vi "ConcatanateFiles.vi"() -> ()   [LabVIEW 2018]
uses:
  <vilib>/Utility/file.llb/Write Delimited Spreadsheet (string).vi
  <vilib>/Utility/file.llb/Read Delimited Spreadsheet (string).vi
panel:
  in  "Combo Box":string(combo)
  in  "path":path=path "C:/RageATE Results/Files to Process"
  out "OutputFile":string="REV-B_TETRA_RX-DVT-Quick_SN_0033_032922-100611_Concat.csv"
  out "Array":string[][](array[string])=[["25", "18.75", "1.000000", "5", "-73", "-1", "-1", "20.000000", "0.577759", "10.832978", "2", "0", "2", "2", "2", "2", "9.995", "10", "-41.21", "31.79", "9.965804", "-39.098881", "-57.496654", "18.397772", "9.965804", "11.713346", "18.311", "0.998", "0.996", "1.807", "3.315", "1.196", "4.993", "3.316", "2.496", "2.516", "3.568", "5.472", "2.824", "2.888", "2.336", "1.448", "0.284", "0.128", "0.686", "0.3", "1.225", "1.12", "24.977425", "25.191151", "27.1", "33", "30.875", "32.25", "31.625", "31.125", "20000", "-41.009443", "136.150678", "1", "0", "3/29/2022 11:45:52 AM", "P0033", "-1", "-1", "adcsync -vADC ERR: 255 255 255 255loop retry_limit_ms 10000...ADC ERR: 255 255 255 255loop retry_limit_ms 9980...ADC ERR: 000 000 000 000ADC ERR: 000 000 000 000ADC ERR: 000 000 000 000ADC ERR: 000 000 000 000ADC ERR: 000 000 000 000ADC ERR: 000 000 000 000ADC ERR: 000 000 000 000ADC ERR: 000 000 000 000ADC0 Frame: 0x30AAA555AAA55500 <- VALIDADC1 Frame: 0x31AAA555AAA55500 <- VALIDADC2 Frame: 0x32AAA555AAA55500 <- VALIDADC3 Frame: 0x33AAA555AAA55500 <- VALIDend retry_limit_ms 9890ADCSYNC PASSED>", "-1", "4F 4F CE CE", "0", "1", "18.000000", "5.000000", "50.000000", "30.000000", "15.000000", "0.000000", "111", "1"], ["25", "18.75", "1.000000", "5", "-73", "-1", "-1", "25.000000", "0.566155", "10.615412", "2", "0", "2", "2", "2", "2", "12.495", "10", "-34.244", "38.756", "9.965804", "-32.195411", "-56.557369", "24.361958", "9.965804", "5.686631", "18.311", "0.997", "0.997", "1.808", "3.317", "1.195", "4.99", "3.316", "2.497", "2.519", "3.56", "5.472", "2.832", "2.888", "2.336", "1.448", "0.29", "0.128", "0.669", "0.291", "1.226", "1.121", "24.97603", "25.195795", "26.05", "33.125", "30.875", "32.125", "31.875", "31.125", "25000", "-41.697643", "10.598856", "2", "1", "3/29/2022 11:46:03 AM", "P0033", "-1", "-1", "-1", "-1", "30 31 32 33", "1", "-1", "18.000000", "5.000000", "50.000000", "30.000000", "8.000000", "0.000000", "111", "1"], ["25", "18.75", "1.000000", "5", "-73", "-1", "-1", "30.000000", "0.56922", "10.672877", "3", "0", "2", "2", "2", "2", "14.995", "10", "-35.696", "37.304", "9.965804", "-33.635349", "-59.768319", "26.13297", "9.965804", "3.927681", "18.311", "0.997", "0.995", "1.807", "3.316", "1.194", "4.992", "3.316", "2.497", "2.516", "3.568", "5.472", "2.824", "2.888", "2.336", "1.448", "0.289", "0.127", "0.689", "0.295", "1.228", "1.155", "24.977425", "25.19043", "28.15", "33", "30.75", "32.375", "31.875", "31.25", "30000", "-42.531268", "11.002014", "3", "1", "3/29/2022 11:46:14 AM", "P0033", "-1", "-1", "-1", "-1", "30 31 32 33", "1", "-1", "18.000000", "5.000000", "50.000000", "30.000000", "6.500000", "0.000000", "111", "1"], ["25", "18.75", "1.000000", "5", "-73", "-1", "-1", "35.000000", "0.567535", "10.641274", "3", "0", "2", "2", "2", "2", "17.495", "10", "-42.928", "30.072", "9.965804", "-40.790008", "-63.593921", "22.803913", "9.965804", "7.334079", "18.329", "0.997", "0.994", "1.807", "3.315", "1.196", "4.992", "3.314", "2.496", "2.516", "3.568", "5.472", "2.824", "2.888", "2.336", "1.448", "0.282", "0.127", "0.684", "0.292", "1.226", "1.117", "24.975447", "25.132133", "27.1", "32.875", "31", "32.375", "31.75", "31.125", "35000", "-41.740204", "10.999033", "4", "1", "3/29/2022 11:46:25 AM", "P0033", "-1", "-1", "-1", "-1", "30 31 32 33", "1", "-1", "18.000000", "5.000000", "50.000000", "30.000000", "9.000000", "0.000000", "111", "1"], ["25", "18.75", "1.000000", "5", "-73", "-1", "-1", "40.000000", "0.559301", "10.486896", "3", "0", "2", "2", "2", "2", "19.995", "10", "-45.764", "27.236", "9.965804", "-43.646918", "-66.38804", "22.741122", "9.965804", "7.37596", "18.32", "0.997", "0.996", "1.808", "3.314", "1.194", "4.989", "3.317", "2.498", "2.516", "3.568", "5.472", "2.832", "2.896", "2.336", "1.456", "0.284", "0.128", "0.657", "0.278", "1.227", "1.141", "24.976114", "25.126818", "26.05", "33.125", "30.75", "32.375", "31.75", "31.25", "40000", "-43.030043", "10.904585", "5", "1", "3/29/2022 11:46:36 AM", "P0033", "-1", "-1", "-1", "-1", "30 31 32 33", "1", "-1", "18.000000", "5.000000", "50.000000", "30.000000", "10.000000", "0.000000", "101", "0"], ["25", "18.75", "2.000000", "5", "-73", "-1", "-1", "20.000000", "0.570127", "10.689885", "2", "0", "2", "2", "2", "2", "9.995", "10", "-39.777", "33.223", "9.965804", "-37.717005", "-57.015434", "19.298429", "9.965804", "10.761566", "18.32", "0.998", "0.995", "1.807", "3.315", "1.196", "4.992", "3.318", "2.496", "2.517", "3.568", "5.472", "2.824", "2.888", "2.336", "1.448", "0.282", "0.128", "0.686", "0.3", "1.226", "1.121", "24.976858", "25.185183", "27.1", "33", "31", "32.375", "31.875", "31.125", "20000", "-41.009443", "14.075206", "6", "1", "3/29/2022 11:46:50 AM", "P0033", "-1", "-1", "-1", "-1", "30 31 32 33", "1", "-1", "18.000000", "5.000000", "50.000000", "30.000000", "15.000000", "0.000000", "111", "1"], ["25", "18.75", "2.000000", "5", "-73", "-1", "-1", "25.000000", "0.566302", "10.618161", "2", "0", "2", "2", "2", "2", "12.495", "10", "-33.63", "39.37", "9.965804", "-31.541197", "-56.658061", "25.116864", "9.965804", "4.971939", "18.311", "0.997", "0.995", "1.807", "3.315", "1.195", "4.992", "3.315", "2.497", "2.517", "3.568", "5.472", "2.832", "2.888", "2.336", "1.448", "0.289", "0.128", "0.669", "0.292", "1.225", "1.123", "24.976875", "25.129929", "27.1", "33", "30.875", "32.375", "32", "31.25", "25000", "-41.697643", "10.478196", "7", "1", "3/29/2022 11:47:00 AM", "P0033", "-1", "-1", "-1", "-1", "30 31 32 33", "1", "-1", "18.000000", "5.000000", "50.000000", "30.000000", "8.000000", "0.000000", "111", "1"], ["25", "18.75", "2.000000", "5", "-73", "-1", "-1", "30.000000", "0.568251", "10.654714", "3", "0", "2", "2", "2", "2", "14.995", "10", "-37.369", "35.631", "9.965804", "-35.334245", "-59.473389", "24.139143", "9.965804", "5.895611", "18.329", "0.996", "0.996", "1.808", "3.314", "1.196", "4.99", "3.317", "2.496", "2.517", "3.568", "5.472", "2.824", "2.888", "2.336", "1.456", "0.282", "0.127", "0.689", "0.295", "1.225", "1.158", "25.036808", "25.127075", "27.1", "32.875", "30.875", "32.25", "31.875", "31.125", "30000", "-42.531268", "11.329658", "8", "1", "3/29/2022 11:47:12 AM", "P0033", "-1", "-1", "-1", "-1", "30 31 32 33", "1", "-1", "18.000000", "5.000000", "50.000000", "30.000000", "6.500000", "0.000000", "111", "1"], ["25", "18.75", "2.000000", "5", "-73", "-1", "-1", "35.000000", "0.56757", "10.641943", "3", "0", "2", "2", "2", "2", "17.495", "10", "-42.834", "30.166", "9.965804", "-40.781149", "-62.504155", "21.723006", "9.965804", "8.329845", "18.311", "0.998", "0.995", "1.807", "3.317", "1.193", "4.99", "3.317", "2.498", "2.517", "3.568", "5.472", "2.832", "2.888", "2.336", "1.448", "0.282", "0.128", "0.684", "0.293", "1.226", "1.128", "24.981291", "25.185307", "27.1", "33.125", "31", "32.375", "32.125", "31.125", "35000", "-41.740204", "11.208919", "9", "1", "3/29/2022 11:47:23 AM", "P0033", "-1", "-1", "-1", "-1", "30 31 32 33", "1", "-1", "18.000000", "5.000000", "50.000000", "30.000000", "9.000000", "0.000000", "111", "1"], ["25", "18.75", "2.000000", "5", "-73", "-1", "-1", "40.000000", "0.55854", "10.472618", "3", "0", "2", "2", "2", "2", "19.995", "10", "-46.104", "26.896", "9.965804", "-44.01646", "-65.539694", "21.523234", "9.965804", "8.564306", "18.329", "0.998", "0.994", "1.807", "3.316", "1.195", "4.992", "3.316", "2.498", "2.517", "3.568", "5.472", "2.832", "2.888", "2.336", "1.456", "0.288", "0.127", "0.657", "0.278", "1.225", "1.132", "24.983986", "25.185158", "26.05", "33.125", "30.875", "32.375", "31.875", "31.25", "40000", "-43.030043", "11.064009", "10", "1", "3/29/2022 11:47:34 AM", "P0033", "-1", "-1", "-1", "-1", "30 31 32 33", "1", "-1", "18.000000", "5.000000", "50.000000", "30.000000", "10.000000", "0.000000", "101", "0"], ["25", "18.75", "3.000000", "5", "-73", "-1", "-1", "20.000000", "0.569196", "10.672434", "2", "0", "2", "2", "2", "2", "9.995", "10", "-41.791", "31.209", "9.965804", "-39.734641", "-57.177492", "17.442851", "9.965804", "12.613508", "18.311", "0.997", "0.996", "1.807", "3.316", "1.195", "4.992", "3.317", "2.498", "2.516", "3.568", "5.472", "2.824", "2.888", "2.336", "1.456", "0.284", "0.128", "0.686", "0.3", "1.227", "1.154", "24.982334", "25.244013", "27.1", "33.125", "31", "32.25", "32", "31.25", "20000", "-41.009443", "13.692614", "11", "1", "3/29/2022 11:47:48 AM", "P0033", "-1", "-1", "-1", "-1", "30 31 32 33", "1", "-1", "18.000000", "5.000000", "50.000000", "30.000000", "15.000000", "0.000000", "111", "1"], ["25", "18.75", "3.000000", "5", "-73", "-1", "-1", "25.000000", "0.565884", "10.610327", "2", "0", "2", "2", "2", "2", "12.495", "10", "-34.544", "38.456", "9.965804", "-32.467577", "-56.90383", "24.436252", "9.965804", "5.64017", "18.311", "0.998", "0.994", "1.807", "3.316", "1.194", "4.99", "3.315", "2.498", "2.518", "3.568", "5.472", "2.832", "2.888", "2.336", "1.448", "0.29", "0.129", "0.668", "0.292", "1.226", "1.149", "24.981443", "25.186216", "27.1", "33.25", "31.125", "32.5", "32", "31.25", "25000", "-41.697643", "10.481807", "12", "1", "3/29/2022 11:47:58 AM", "P0033", "-1", "-1", "-1", "-1", "30 31 32 33", "1", "-1", "18.000000", "5.000000", "50.000000", "30.000000", "8.000000", "0.000000", "111", "1"], ["25", "18.75", "3.000000", "5", "-73", "-1", "-1", "30.000000", "0.568936", "10.667548", "3", "0", "2", "2", "2", "2", "14.995", "10", "-36.579", "36.421", "9.965804", "-34.529812", "-59.478393", "24.948581", "9.965804", "5.100607", "18.32", "0.997", "0.996", "1.808", "3.318", "1.194", "4.99", "3.316", "2.497", "2.517", "3.568", "5.472", "2.824", "2.888", "2.336", "1.448", "0.288", "0.128", "0.689", "0.295", "1.226", "1.147", "24.978163", "25.18915", "28.15", "33", "31", "32.25", "32", "31.25", "30000", "-42.531268", "10.500729", "13", "1", "3/29/2022 11:48:09 AM", "P0033", "-1", "-1", "-1", "-1", "30 31 32 33", "1", "-1", "18.000000", "5.000000", "50.000000", "30.000000", "6.500000", "0.000000", "111", "1"], ["25", "18.75", "3.000000", "5", "-73", "-1", "-1", "35.000000", "0.566788", "10.627281", "3", "0", "2", "2", "2", "2", "17.495", "10", "-43.405", "29.595", "9.965804", "-41.22646", "-63.599396", "22.372936", "9.965804", "7.805604", "18.32", "0.996", "0.995", "1.807", "3.315", "1.195", "4.993", "3.314", "2.497", "2.515", "3.568", "5.472", "2.824", "2.888", "2.336", "1.448", "0.284", "0.127", "0.684", "0.292", "1.226", "1.112", "24.98241", "25.189056", "28.15", "33.125", "31.125", "32.5", "32", "31.375", "35000", "-41.740204", "10.705545", "14", "1", "3/29/2022 11:48:19 AM", "P0033", "-1", "-1", "-1", "-1", "30 31 32 33", "1", "-1", "18.000000", "5.000000", "50.000000", "30.000000", "9.000000", "0.000000", "101", "0"], ["25", "18.75", "3.000000", "5", "-73", "-1", "-1", "40.000000", "0.559835", "10.496908", "3", "0", "2", "2", "2", "2", "19.995", "10", "-45.892", "27.108", "9.965804", "-43.715005", "-66.201275", "22.486271", "9.965804", "7.690725", "18.329", "0.998", "0.995", "1.808", "3.315", "1.195", "4.99", "3.316", "2.499", "2.516", "3.568", "5.472", "2.832", "2.896", "2.336", "1.448", "0.282", "0.129", "0.657", "0.278", "1.226", "1.119", "25.036692", "25.130362", "27.1", "33", "31", "32.375", "32", "31.25", "40000", "-43.030043", "10.748362", "15", "1", "3/29/2022 11:48:30 AM", "P0033", "-1", "-1", "-1", "-1", "30 31 32 33", "1", "-1", "18.000000", "5.000000", "50.000000", "30.000000", "10.000000", "0.000000", "101", "0"], ["25", "18.75", "4.000000", "5", "-73", "-1", "-1", "20.000000", "0.569984", "10.687207", "2", "0", "2", "2", "2", "2", "9.995", "10", "-40.021", "32.979", "9.965804", "-37.912785", "-56.529531", "18.616746", "9.965804", "11.491469", "18.293", "0.996", "0.996", "1.807", "3.316", "1.193", "4.992", "3.317", "2.496", "2.516", "3.568", "5.472", "2.824", "2.888", "2.336", "1.448", "0.289", "0.127", "0.686", "0.3", "1.226", "1.122", "25.093027", "25.250462", "27.1", "33.25", "31", "32.5", "32.25", "31.125", "20000", "-41.009443", "13.610743", "16", "1", "3/29/2022 11:48:44 AM", "P0033", "-1", "-1", "-1", "-1", "30 31 32 33", "1", "-1", "18.000000", "5.000000", "50.000000", "30.000000", "15.000000", "0.000000", "111", "1"], ["25", "18.75", "4.000000", "5", "-73", "-1", "-1", "25.000000", "0.565701", "10.60689", "2", "0", "2", "2", "2", "2", "12.495", "10", "-33.558", "39.442", "9.965804", "-31.453021", "-56.199732", "24.746711", "9.965804", "5.358268", "18.32", "0.999", "0.996", "1.809", "3.316", "1.196", "4.99", "3.317", "2.497", "2.517", "3.568", "5.472", "2.832", "2.888", "2.336", "1.448", "0.282", "0.128", "0.669", "0.292", "1.226", "1.125", "25.034227", "25.191473", "27.1", "33.125", "31.125", "32.5", "32.125", "31.375", "25000", "-41.697643", "10.32326", "17", "1", "3/29/2022 11:48:54 AM", "P0033", "-1", "-1", "-1", "-1", "30 31 32 33", "1", "-1", "18.000000", "5.000000", "50.000000", "30.000000", "8.000000", "0.000000", "111", "1"], ["25", "18.75", "4.000000", "5", "-73", "-1", "-1", "30.000000", "0.569667", "10.681251", "3", "0", "2", "2", "2", "2", "14.995", "10", "-36.871", "36.129", "9.965804", "-34.816471", "-59.611387", "24.794916", "9.965804", "5.259613", "18.311", "0.996", "0.995", "1.807", "3.315", "1.196", "4.99", "3.317", "2.496", "2.516", "3.568", "5.472", "2.824", "2.888", "2.336", "1.448", "0.29", "0.128", "0.688", "0.295", "1.226", "1.135", "25.033773", "25.189878", "28.15", "33.125", "31.125", "32.375", "32.125", "31.25", "30000", "-42.531268", "10.356341", "18", "1", "3/29/2022 11:49:04 AM", "P0033", "-1", "-1", "-1", "-1", "30 31 32 33", "1", "-1", "18.000000", "5.000000", "50.000000", "30.000000", "6.500000", "0.000000", "111", "1"], ["25", "18.75", "4.000000", "5", "-73", "-1", "-1", "35.000000", "0.567024", "10.631707", "3", "0", "2", "2", "2", "2", "17.495", "10", "-42.439", "30.561", "9.965804", "-40.275433", "-63.414415", "23.138982", "9.965804", "7.024585", "18.311", "0.997", "0.994", "1.807", "3.314", "1.195", "4.99", "3.317", "2.496", "2.517", "3.568", "5.472", "2.832", "2.888", "2.336", "1.456", "0.288", "0.128", "0.683", "0.293", "1.225", "1.12", "25.08617", "25.183359", "27.1", "33.125", "31.125", "32.375", "32", "31.375", "35000", "-41.740204", "10.898454", "19", "1", "3/29/2022 11:49:15 AM", "P0033", "-1", "-1", "-1", "-1", "30 31 32 33", "1", "-1", "18.000000", "5.000000", "50.000000", "30.000000", "9.000000", "0.000000", "111", "1"], ["25", "18.75", "4.000000", "5", "-73", "-1", "-1", "40.000000", "0.558596", "10.473666", "3", "0", "2", "2", "2", "2", "19.995", "10", "-45.617", "27.383", "9.965804", "-43.461601", "-65.824684", "22.363083", "9.965804", "7.792316", "18.329", "0.997", "0.996", "1.808", "3.315", "1.194", "4.992", "3.315", "2.498", "2.516", "3.568", "5.472", "2.832", "2.896", "2.336", "1.456", "0.288", "0.128", "0.657", "0.278", "1.225", "1.109", "25.031197", "25.187513", "27.1", "33.125", "31", "32.5", "32", "31.375", "40000", "-43.030043", "10.286318", "20", "1", "3/29/2022 11:49:26 AM", "P0033", "-1", "-1", "-1", "-1", "30 31 32 33", "1", "-1", "18.000000", "5.000000", "50.000000", "30.000000", "10.000000", "0.000000", "101", "0"], ["25", "18.75", "5.000000", "5", "-73", "-1", "-1", "20.000000", "0.568759", "10.664233", "2", "0", "2", "2", "2", "2", "9.995", "10", "-40.401", "32.599", "9.965804", "-38.239629", "-56.65276", "18.413131", "9.965804", "11.74824", "18.311", "0.997", "0.995", "1.807", "3.315", "1.195", "4.992", "3.316", "2.498", "2.516", "3.568", "5.472", "2.824", "2.888", "2.336", "1.456", "0.288", "0.128", "0.686", "0.3", "1.225", "1.149", "24.959276", "25.241495", "27.1", "33", "31.125", "32.5", "32.125", "31.125", "20000", "-41.009443", "13.582175", "21", "1", "3/29/2022 11:49:39 AM", "P0033", "-1", "-1", "-1", "-1", "30 31 32 33", "1", "-1", "18.000000", "5.000000", "50.000000", "30.000000", "15.000000", "0.000000", "111", "1"], ["25", "18.75", "5.000000", "5", "-73", "-1", "-1", "25.000000", "0.564387", "10.582251", "2", "0", "2", "2", "2", "2", "12.495", "10", "-34.486", "38.514", "9.965804", "-32.495831", "-56.909748", "24.413917", "9.965804", "5.576252", "18.32", "0.998", "0.994", "1.807", "3.316", "1.193", "4.992", "3.316", "2.498", "2.516", "3.568", "5.472", "2.832", "2.888", "2.336", "1.448", "0.282", "0.128", "0.669", "0.292", "1.225", "1.139", "25.023981", "25.185495", "27.1", "33.25", "31.125", "32.5", "32", "31.25", "25000", "-41.697643", "10.338612", "22", "1", "3/29/2022 11:49:50 AM", "P0033", "-1", "-1", "-1", "-1", "30 31 32 33", "1", "-1", "18.000000", "5.000000", "50.000000", "30.000000", "8.000000", "0.000000", "111", "1"], ["25", "18.75", "5.000000", "5", "-73", "-1", "-1", "30.000000", "0.568503", "10.659439", "3", "0", "2", "2", "2", "2", "14.995", "10", "-36.257", "36.743", "9.965804", "-34.227624", "-59.03033", "24.802706", "9.965804", "5.22667", "18.311", "0.997", "0.995", "1.808", "3.316", "1.195", "4.99", "3.316", "2.497", "2.516", "3.568", "5.472", "2.824", "2.888", "2.336", "1.448", "0.282", "0.128", "0.689", "0.294", "1.226", "1.113", "25.015224", "25.179966", "28.15", "33.25", "31.25", "32.5", "32.125", "31.25", "30000", "-42.531268", "10.3116", "23", "1", "3/29/2022 11:50:00 AM", "P0033", "-1", "-1", "-1", "-1", "30 31 32 33", "1", "-1", "18.000000", "5.000000", "50.000000", "30.000000", "6.500000", "0.000000", "111", "1"], ["25", "18.75", "5.000000", "5", "-73", "-1", "-1", "35.000000", "0.566003", "10.612558", "3", "0", "2", "2", "2", "2", "17.495", "10", "-42.197", "30.803", "9.965804", "-40.042527", "-62.132186", "22.089659", "9.965804", "8.064814", "18.311", "0.998", "0.996", "1.807", "3.315", "1.195", "4.992", "3.316", "2.496", "2.517", "3.568", "5.472", "2.824", "2.888", "2.336", "1.456", "0.288", "0.128", "0.684", "0.292", "1.226", "1.145", "25.013937", "25.181458", "28.15", "33.25", "31.25", "32.375", "32.125", "31.25", "35000", "-41.740204", "10.377699", "24", "1", "3/29/2022 11:50:10 AM", "P0033", "-1", "-1", "-1", "-1", "30 31 32 33", "1", "-1", "18.000000", "5.000000", "50.000000", "30.000000", "9.000000", "0.000000", "111", "1"], ["25", "18.75", "5.000000", "5", "-73", "-1", "-1", "40.000000", "0.558588", "10.473525", "3", "0", "2", "2", "2", "2", "19.995", "10", "-45.624", "27.376", "9.965804", "-43.466521", "-65.070224", "21.603703", "9.965804", "8.553776", "18.311", "0.996", "0.994", "1.807", "3.315", "1.194", "4.989", "3.315", "2.498", "2.518", "3.568", "5.472", "2.832", "2.888", "2.336", "1.456", "0.282", "0.128", "0.657", "0.278", "1.225", "1.135", "25.010406", "25.240318", "26.05", "33.25", "31", "32.5", "32.125", "31.375", "40000", "-43.030043", "10.290322", "25", "1", "3/29/2022 11:50:21 AM", "P0033", "-1", "-1", "-1", "-1", "30 31 32 33", "1", "-1", "18.000000", "5.000000", "50.000000", "30.000000", "10.000000", "0.000000", "101", "0"], ["25", "18.75", "6.000000", "5", "-73", "-1", "-1", "20.000000", "0.567979", "10.649612", "2", "0", "2", "2", "2", "2", "9.995", "10", "-39.876", "33.124", "9.965804", "-37.689382", "-56.766567", "19.077185", "9.965804", "11.109433", "18.32", "0.996", "0.996", "1.808", "3.317", "1.196", "4.99", "3.314", "2.496", "2.517", "3.568", "5.472", "2.824", "2.888", "2.336", "1.456", "0.284", "0.128", "0.685", "0.3", "1.225", "1.136", "25.006052", "25.180799", "28.15", "33.125", "31.125", "32.5", "32.25", "31.375", "20000", "-41.009443", "13.656313", "26", "1", "3/29/2022 11:50:34 AM", "P0033", "-1", "-1", "-1", "-1", "30 31 32 33", "1", "-1", "18.000000", "5.000000", "50.000000", "30.000000", "15.000000", "0.000000", "111", "1"], ["25", "18.75", "6.000000", "5", "-73", "-1", "-1", "25.000000", "0.56491", "10.592068", "2", "0", "2", "2", "2", "2", "12.495", "10", "-34.01", "38.99", "9.965804", "-31.871954", "-55.985571", "24.113616", "9.965804", "6.024429", "18.329", "0.996", "0.994", "1.807", "3.315", "1.193", "4.993", "3.317", "2.496", "2.516", "3.568", "5.472", "2.832", "2.888", "2.336", "1.448", "0.284", "0.128", "0.668", "0.292", "1.225", "1.113", "25.014597", "25.185217", "27.1", "33.375", "31.25", "32.5", "32.125", "31.375", "25000", "-41.697643", "10.37923", "27", "1", "3/29/2022 11:50:45 AM", "P0033", "-1", "-1", "-1", "-1", "30 31 32 33", "1", "-1", "18.000000", "5.000000", "50.000000", "30.000000", "8.000000", "0.000000", "111", "1"], ["25", "18.75", "6.000000", "5", "-73", "-1", "-1", "30.000000", "0.567354", "10.637895", "3", "0", "2", "2", "2", "2", "14.995", "10", "-37.283", "35.717", "9.965804", "-35.186326", "-60.015322", "24.828996", "9.965804", "5.267678", "18.32", "0.996", "0.996", "1.808", "3.315", "1.195", "4.992", "3.317", "2.498", "2.517", "3.568", "5.472", "2.824", "2.888", "2.336", "1.448", "0.29", "0.129", "0.688", "0.295", "1.226", "1.106", "25.006163", "25.179977", "28.15", "33.25", "31", "32.5", "32.25", "31.25", "30000", "-42.531268", "10.365277", "28", "1", "3/29/2022 11:50:55 AM", "P0033", "-1", "-1", "-1", "-1", "30 31 32 33", "1", "-1", "18.000000", "5.000000", "50.000000", "30.000000", "6.500000", "0.000000", "111", "1"], ["25", "18.75", "6.000000", "5", "-73", "-1", "-1", "35.000000", "0.565674", "10.60638", "3", "0", "2", "2", "2", "2", "17.495", "10", "-41.248", "31.752", "9.965804", "-38.992964", "-62.000115", "23.007151", "9.965804", "7.247885", "18.311", "0.997", "0.994", "1.807", "3.315", "1.194", "4.99", "3.317", "2.497", "2.518", "3.568", "5.472", "2.832", "2.888", "2.336", "1.456", "0.284", "0.129", "0.683", "0.292", "1.224", "1.115", "24.951511", "25.182125", "28.15", "33.25", "31.125", "32.625", "32", "31.375", "35000", "-41.740204", "10.28063", "29", "1", "3/29/2022 11:51:05 AM", "P0033", "-1", "-1", "-1", "-1", "30 31 32 33", "1", "-1", "18.000000", "5.000000", "50.000000", "30.000000", "9.000000", "0.000000", "111", "1"], ["25", "18.75", "6.000000", "5", "-73", "-1", "-1", "40.000000", "0.559541", "10.491401", "3", "0", "2", "2", "2", "2", "19.995", "10", "-45.525", "27.475", "9.965804", "-43.40969", "-64.476696", "21.067006", "9.965804", "9.048304", "18.329", "0.996", "0.996", "1.807", "3.316", "1.195", "4.992", "3.317", "2.498", "2.515", "3.568", "5.472", "2.832", "2.896", "2.336", "1.456", "0.288", "0.128", "0.657", "0.279", "1.225", "1.117", "24.952892", "25.180176", "26.05", "33.25", "31", "32.5", "32.125", "31.25", "40000", "-43.030043", "10.361334", "30", "1", "3/29/2022 11:51:16 AM", "P0033", "-1", "-1", "-1", "-1", "30 31 32 33", "1", "-1", "18.000000", "5.000000", "50.000000", "30.000000", "10.000000", "0.000000", "101", "0"], ["25", "18.75", "7.000000", "5", "-73", "-1", "-1", "20.000000", "0.569671", "10.681324", "2", "0", "2", "2", "2", "2", "9.995", "10", "-40.815", "32.185", "9.965804", "-38.665384", "-56.780314", "18.11493", "9.965804", "12.034686", "18.311", "0.996", "0.996", "1.807", "3.316", "1.195", "4.995", "3.314", "2.496", "2.518", "3.568", "5.472", "2.824", "2.888", "2.336", "1.448", "0.282", "0.127", "0.686", "0.3", "1.226", "1.127", "24.953074", "25.179266", "27.1", "33.375", "31.25", "32.375", "32.25", "31.25", "20000", "-41.009443", "13.584268", "31", "1", "3/29/2022 11:51:29 AM", "P0033", "-1", "-1", "-1", "-1", "30 31 32 33", "1", "-1", "18.000000", "5.000000", "50.000000", "30.000000", "15.000000", "0.000000", "111", "1"], ["25", "18.75", "7.000000", "5", "-73", "-1", "-1", "25.000000", "0.565739", "10.607599", "2", "0", "2", "2", "2", "2", "12.495", "10", "-35.054", "37.946", "9.965804", "-33.063722", "-57.302932", "24.23921", "9.965804", "5.751068", "18.32", "0.996", "0.996", "1.807", "3.316", "1.195", "4.992", "3.316", "2.498", "2.516", "3.568", "5.472", "2.832", "2.888", "2.336", "1.456", "0.288", "0.128", "0.669", "0.292", "1.228", "1.159", "24.952223", "25.229593", "27.1", "33.25", "31.25", "32.625", "32.125", "31.375", "25000", "-41.697643", "10.307795", "32", "1", "3/29/2022 11:51:40 AM", "P0033", "-1", "-1", "-1", "-1", "30 31 32 33", "1", "-1", "18.000000", "5.000000", "50.000000", "30.000000", "8.000000", "0.000000", "111", "1"], ["25", "18.75", "7.000000", "5", "-73", "-1", "-1", "30.000000", "0.568261", "10.654898", "3", "0", "2", "2", "2", "2", "14.995", "10", "-36.264", "36.736", "9.965804", "-34.133015", "-59.415787", "25.282772", "9.965804", "4.848213", "18.329", "0.997", "0.996", "1.807", "3.314", "1.194", "4.99", "3.317", "2.496", "2.516", "3.568", "5.472", "2.824", "2.888", "2.336", "1.448", "0.283", "0.128", "0.689", "0.295", "1.225", "1.117", "24.950842", "25.228264", "28.15", "33.25", "31.125", "32.625", "32.125", "31.375", "30000", "-42.531268", "10.490804", "33", "1", "3/29/2022 11:51:50 AM", "P0033", "-1", "-1", "-1", "-1", "30 31 32 33", "1", "-1", "18.000000", "5.000000", "50.000000", "30.000000", "6.500000", "0.000000", "111", "1"], ["25", "18.75", "7.000000", "5", "-73", "-1", "-1", "35.000000", "0.567675", "10.643908", "3", "0", "2", "2", "2", "2", "17.495", "10", "-42.534", "30.466", "9.965804", "-40.439073", "-63.069629", "22.630556", "9.965804", "7.464371", "18.311", "0.996", "0.995", "1.807", "3.315", "1.195", "4.99", "3.315", "2.496", "2.516", "3.568", "5.472", "2.824", "2.888", "2.336", "1.448", "0.288", "0.128", "0.684", "0.292", "1.226", "1.114", "24.896477", "25.16938", "27.1", "33.25", "31.25", "32.625", "32.125", "31.375", "35000", "-41.740204", "10.569302", "34", "1", "3/29/2022 11:52:01 AM", "P0033", "-1", "-1", "-1", "-1", "30 31 32 33", "1", "-1", "18.000000", "5.000000", "50.000000", "30.000000", "9.000000", "0.000000", "111", "1"], ["25", "18.75", "7.000000", "5", "-73", "-1", "-1", "40.000000", "0.559448", "10.489652", "3", "0", "2", "2", "2", "2", "19.995", "10", "-46.551", "26.449", "9.965804", "-44.613001", "-66.004291", "21.39129", "9.965804", "8.546709", "18.329", "0.997", "0.996", "1.807", "3.316", "1.194", "4.993", "3.315", "2.497", "2.516", "3.568", "5.472", "2.832", "2.888", "2.336", "1.456", "0.282", "0.127", "0.657", "0.278", "1.225", "1.136", "24.957314", "25.16938", "27.1", "33.125", "31.125", "32.625", "31.875", "31.375", "40000", "-43.030043", "10.409809", "35", "1", "3/29/2022 11:52:11 AM", "P0033", "-1", "-1", "-1", "-1", "30 31 32 33", "1", "-1", "18.000000", "5.000000", "50.000000", "30.000000", "10.000000", "0.000000", "101", "0"], ["25", "18.75", "8.000000", "5", "-73", "-1", "-1", "20.000000", "0.568566", "10.660607", "2", "0", "2", "2", "2", "2", "9.995", "10", "-40.849", "32.151", "9.965804", "-38.818566", "-56.347075", "17.528509", "9.965804", "12.501925", "18.311", "0.998", "0.995", "1.807", "3.315", "1.195", "4.992", "3.315", "2.496", "2.516", "3.568", "5.472", "2.824", "2.888", "2.336", "1.448", "0.284", "0.128", "0.686", "0.3", "1.226", "1.117", "25.019802", "25.228247", "27.1", "33.25", "31.125", "32.625", "32.125", "31.375", "20000", "-41.009443", "13.716725", "36", "1", "3/29/2022 11:52:25 AM", "P0033", "-1", "-1", "-1", "-1", "30 31 32 33", "1", "-1", "18.000000", "5.000000", "50.000000", "30.000000", "15.000000", "0.000000", "111", "1"], ["25", "18.75", "8.000000", "5", "-73", "-1", "-1", "25.000000", "0.565711", "10.607083", "2", "0", "2", "2", "2", "2", "12.495", "10", "-34.8", "38.2", "9.965804", "-32.769672", "-57.008907", "24.239235", "9.965804", "5.791093", "18.329", "0.997", "0.995", "1.807", "3.314", "1.194", "4.993", "3.317", "2.496", "2.516", "3.568", "5.472", "2.832", "2.888", "2.336", "1.448", "0.282", "0.128", "0.669", "0.292", "1.228", "1.128", "25.022074", "25.22739", "27.1", "33.25", "31.25", "32.625", "32", "31.25", "25000", "-41.697643", "10.948414", "37", "1", "3/29/2022 11:52:36 AM", "P0033", "-1", "-1", "-1", "-1", "30 31 32 33", "1", "-1", "18.000000", "5.000000", "50.000000", "30.000000", "8.000000", "0.000000", "111", "1"], ["25", "18.75", "8.000000", "5", "-73", "-1", "-1", "30.000000", "0.569299", "10.674366", "3", "0", "2", "2", "2", "2", "14.995", "10", "-36.661", "36.339", "9.965804", "-34.535792", "-59.050958", "24.515167", "9.965804", "5.610042", "18.302", "0.998", "0.995", "1.807", "3.316", "1.195", "4.989", "3.314", "2.498", "2.515", "3.568", "5.472", "2.824", "2.888", "2.336", "1.456", "0.29", "0.128", "0.688", "0.295", "1.226", "1.114", "25.021591", "25.230801", "28.15", "33.375", "31.25", "32.5", "32.25", "31.5", "30000", "-42.531268", "10.472914", "38", "1", "3/29/2022 11:52:46 AM", "P0033", "-1", "-1", "-1", "-1", "30 31 32 33", "1", "-1", "18.000000", "5.000000", "50.000000", "30.000000", "6.500000", "0.000000", "111", "1"], ["25", "18.75", "8.000000", "5", "-73", "-1", "-1", "35.000000", "0.566667", "10.625016", "3", "0", "2", "2", "2", "2", "17.495", "10", "-43.481", "29.519", "9.965804", "-41.42763", "-63.649674", "22.222044", "9.965804", "7.831326", "18.32", "0.996", "0.996", "1.806", "3.314", "1.195", "4.993", "3.315", "2.497", "2.516", "3.568", "5.472", "2.824", "2.888", "2.336", "1.448", "0.284", "0.128", "0.684", "0.292", "1.225", "1.108", "25.019392", "25.230145", "28.15", "33.125", "31.25", "32.625", "32.25", "31.375", "35000", "-41.740204", "10.598635", "39", "1", "3/29/2022 11:52:57 AM", "P0033", "-1", "-1", "-1", "-1", "30 31 32 33", "1", "-1", "18.000000", "5.000000", "50.000000", "30.000000", "9.000000", "0.000000", "101", "0"], ["25", "18.75", "8.000000", "5", "-73", "-1", "-1", "40.000000", "0.558543", "10.472679", "3", "0", "2", "2", "2", "2", "19.995", "10", "-46.351", "26.649", "9.965804", "-44.220796", "-65.350936", "21.13014", "9.965804", "9.000064", "18.32", "0.996", "0.995", "1.807", "3.315", "1.195", "4.99", "3.317", "2.497", "2.517", "3.568", "5.472", "2.832", "2.896", "2.336", "1.456", "0.284", "0.128", "0.657", "0.278", "1.224", "1.101", "25.08005", "25.225355", "27.1", "33.375", "31", "32.5", "32.125", "31.375", "40000", "-43.030043", "10.739114", "40", "1", "3/29/2022 11:53:08 AM", "P0033", "-1", "-1", "-1", "-1", "30 31 32 33", "1", "-1", "18.000000", "5.000000", "50.000000", "30.000000", "10.000000", "0.000000", "101", "0"]]
  out "subarray":string[][](array[string])=[["25", "18.75", "1.000000", "5", "-73", "-1", "-1", "20.000000", "0.577759", "10.832978", "2", "0", "2", "2", "2", "2", "9.995", "10", "-41.21", "31.79", "9.965804", "-39.098881", "-57.496654", "18.397772", "9.965804", "11.713346", "18.311", "0.998", "0.996", "1.807", "3.315", "1.196", "4.993", "3.316", "2.496", "2.516", "3.568", "5.472", "2.824", "2.888", "2.336", "1.448", "0.284", "0.128", "0.686", "0.3", "1.225", "1.12", "24.977425", "25.191151", "27.1", "33", "30.875", "32.25", "31.625", "31.125", "20000", "-41.009443", "136.150678", "1", "0", "3/29/2022 11:45:52 AM", "P0033", "-1", "-1", "adcsync -vADC ERR: 255 255 255 255loop retry_limit_ms 10000...ADC ERR: 255 255 255 255loop retry_limit_ms 9980...ADC ERR: 000 000 000 000ADC ERR: 000 000 000 000ADC ERR: 000 000 000 000ADC ERR: 000 000 000 000ADC ERR: 000 000 000 000ADC ERR: 000 000 000 000ADC ERR: 000 000 000 000ADC ERR: 000 000 000 000ADC0 Frame: 0x30AAA555AAA55500 <- VALIDADC1 Frame: 0x31AAA555AAA55500 <- VALIDADC2 Frame: 0x32AAA555AAA55500 <- VALIDADC3 Frame: 0x33AAA555AAA55500 <- VALIDend retry_limit_ms 9890ADCSYNC PASSED>", "-1", "4F 4F CE CE", "0", "1", "18.000000", "5.000000", "50.000000", "30.000000", "15.000000", "0.000000", "111", "1", "9", "REV-B_TETRA_RX-DVT-Quick_SN_P0033_032922-114225.csv"], ["25", "18.75", "1.000000", "5", "-73", "-1", "-1", "25.000000", "0.566155", "10.615412", "2", "0", "2", "2", "2", "2", "12.495", "10", "-34.244", "38.756", "9.965804", "-32.195411", "-56.557369", "24.361958", "9.965804", "5.686631", "18.311", "0.997", "0.997", "1.808", "3.317", "1.195", "4.99", "3.316", "2.497", "2.519", "3.56", "5.472", "2.832", "2.888", "2.336", "1.448", "0.29", "0.128", "0.669", "0.291", "1.226", "1.121", "24.97603", "25.195795", "26.05", "33.125", "30.875", "32.125", "31.875", "31.125", "25000", "-41.697643", "10.598856", "2", "1", "3/29/2022 11:46:03 AM", "P0033", "-1", "-1", "-1", "-1", "30 31 32 33", "1", "-1", "18.000000", "5.000000", "50.000000", "30.000000", "8.000000", "0.000000", "111", "1", "9", "REV-B_TETRA_RX-DVT-Quick_SN_P0033_032922-114225.csv"], ["25", "18.75", "1.000000", "5", "-73", "-1", "-1", "30.000000", "0.56922", "10.672877", "3", "0", "2", "2", "2", "2", "14.995", "10", "-35.696", "37.304", "9.965804", "-33.635349", "-59.768319", "26.13297", "9.965804", "3.927681", "18.311", "0.997", "0.995", "1.807", "3.316", "1.194", "4.992", "3.316", "2.497", "2.516", "3.568", "5.472", "2.824", "2.888", "2.336", "1.448", "0.289", "0.127", "0.689", "0.295", "1.228", "1.155", "24.977425", "25.19043", "28.15", "33", "30.75", "32.375", "31.875", "31.25", "30000", "-42.531268", "11.002014", "3", "1", "3/29/2022 11:46:14 AM", "P0033", "-1", "-1", "-1", "-1", "30 31 32 33", "1", "-1", "18.000000", "5.000000", "50.000000", "30.000000", "6.500000", "0.000000", "111", "1", "9", "REV-B_TETRA_RX-DVT-Quick_SN_P0033_032922-114225.csv"], ["25", "18.75", "1.000000", "5", "-73", "-1", "-1", "35.000000", "0.567535", "10.641274", "3", "0", "2", "2", "2", "2", "17.495", "10", "-42.928", "30.072", "9.965804", "-40.790008", "-63.593921", "22.803913", "9.965804", "7.334079", "18.329", "0.997", "0.994", "1.807", "3.315", "1.196", "4.992", "3.314", "2.496", "2.516", "3.568", "5.472", "2.824", "2.888", "2.336", "1.448", "0.282", "0.127", "0.684", "0.292", "1.226", "1.117", "24.975447", "25.132133", "27.1", "32.875", "31", "32.375", "31.75", "31.125", "35000", "-41.740204", "10.999033", "4", "1", "3/29/2022 11:46:25 AM", "P0033", "-1", "-1", "-1", "-1", "30 31 32 33", "1", "-1", "18.000000", "5.000000", "50.000000", "30.000000", "9.000000", "0.000000", "111", "1", "9", "REV-B_TETRA_RX-DVT-Quick_SN_P0033_032922-114225.csv"], ["25", "18.75", "1.000000", "5", "-73", "-1", "-1", "40.000000", "0.559301", "10.486896", "3", "0", "2", "2", "2", "2", "19.995", "10", "-45.764", "27.236", "9.965804", "-43.646918", "-66.38804", "22.741122", "9.965804", "7.37596", "18.32", "0.997", "0.996", "1.808", "3.314", "1.194", "4.989", "3.317", "2.498", "2.516", "3.568", "5.472", "2.832", "2.896", "2.336", "1.456", "0.284", "0.128", "0.657", "0.278", "1.227", "1.141", "24.976114", "25.126818", "26.05", "33.125", "30.75", "32.375", "31.75", "31.25", "40000", "-43.030043", "10.904585", "5", "1", "3/29/2022 11:46:36 AM", "P0033", "-1", "-1", "-1", "-1", "30 31 32 33", "1", "-1", "18.000000", "5.000000", "50.000000", "30.000000", "10.000000", "0.000000", "101", "0", "9", "REV-B_TETRA_RX-DVT-Quick_SN_P0033_032922-114225.csv"], ["25", "18.75", "2.000000", "5", "-73", "-1", "-1", "20.000000", "0.570127", "10.689885", "2", "0", "2", "2", "2", "2", "9.995", "10", "-39.777", "33.223", "9.965804", "-37.717005", "-57.015434", "19.298429", "9.965804", "10.761566", "18.32", "0.998", "0.995", "1.807", "3.315", "1.196", "4.992", "3.318", "2.496", "2.517", "3.568", "5.472", "2.824", "2.888", "2.336", "1.448", "0.282", "0.128", "0.686", "0.3", "1.226", "1.121", "24.976858", "25.185183", "27.1", "33", "31", "32.375", "31.875", "31.125", "20000", "-41.009443", "14.075206", "6", "1", "3/29/2022 11:46:50 AM", "P0033", "-1", "-1", "-1", "-1", "30 31 32 33", "1", "-1", "18.000000", "5.000000", "50.000000", "30.000000", "15.000000", "0.000000", "111", "1", "9", "REV-B_TETRA_RX-DVT-Quick_SN_P0033_032922-114225.csv"], ["25", "18.75", "2.000000", "5", "-73", "-1", "-1", "25.000000", "0.566302", "10.618161", "2", "0", "2", "2", "2", "2", "12.495", "10", "-33.63", "39.37", "9.965804", "-31.541197", "-56.658061", "25.116864", "9.965804", "4.971939", "18.311", "0.997", "0.995", "1.807", "3.315", "1.195", "4.992", "3.315", "2.497", "2.517", "3.568", "5.472", "2.832", "2.888", "2.336", "1.448", "0.289", "0.128", "0.669", "0.292", "1.225", "1.123", "24.976875", "25.129929", "27.1", "33", "30.875", "32.375", "32", "31.25", "25000", "-41.697643", "10.478196", "7", "1", "3/29/2022 11:47:00 AM", "P0033", "-1", "-1", "-1", "-1", "30 31 32 33", "1", "-1", "18.000000", "5.000000", "50.000000", "30.000000", "8.000000", "0.000000", "111", "1", "9", "REV-B_TETRA_RX-DVT-Quick_SN_P0033_032922-114225.csv"], ["25", "18.75", "2.000000", "5", "-73", "-1", "-1", "30.000000", "0.568251", "10.654714", "3", "0", "2", "2", "2", "2", "14.995", "10", "-37.369", "35.631", "9.965804", "-35.334245", "-59.473389", "24.139143", "9.965804", "5.895611", "18.329", "0.996", "0.996", "1.808", "3.314", "1.196", "4.99", "3.317", "2.496", "2.517", "3.568", "5.472", "2.824", "2.888", "2.336", "1.456", "0.282", "0.127", "0.689", "0.295", "1.225", "1.158", "25.036808", "25.127075", "27.1", "32.875", "30.875", "32.25", "31.875", "31.125", "30000", "-42.531268", "11.329658", "8", "1", "3/29/2022 11:47:12 AM", "P0033", "-1", "-1", "-1", "-1", "30 31 32 33", "1", "-1", "18.000000", "5.000000", "50.000000", "30.000000", "6.500000", "0.000000", "111", "1", "9", "REV-B_TETRA_RX-DVT-Quick_SN_P0033_032922-114225.csv"], ["25", "18.75", "2.000000", "5", "-73", "-1", "-1", "35.000000", "0.56757", "10.641943", "3", "0", "2", "2", "2", "2", "17.495", "10", "-42.834", "30.166", "9.965804", "-40.781149", "-62.504155", "21.723006", "9.965804", "8.329845", "18.311", "0.998", "0.995", "1.807", "3.317", "1.193", "4.99", "3.317", "2.498", "2.517", "3.568", "5.472", "2.832", "2.888", "2.336", "1.448", "0.282", "0.128", "0.684", "0.293", "1.226", "1.128", "24.981291", "25.185307", "27.1", "33.125", "31", "32.375", "32.125", "31.125", "35000", "-41.740204", "11.208919", "9", "1", "3/29/2022 11:47:23 AM", "P0033", "-1", "-1", "-1", "-1", "30 31 32 33", "1", "-1", "18.000000", "5.000000", "50.000000", "30.000000", "9.000000", "0.000000", "111", "1", "9", "REV-B_TETRA_RX-DVT-Quick_SN_P0033_032922-114225.csv"], ["25", "18.75", "2.000000", "5", "-73", "-1", "-1", "40.000000", "0.55854", "10.472618", "3", "0", "2", "2", "2", "2", "19.995", "10", "-46.104", "26.896", "9.965804", "-44.01646", "-65.539694", "21.523234", "9.965804", "8.564306", "18.329", "0.998", "0.994", "1.807", "3.316", "1.195", "4.992", "3.316", "2.498", "2.517", "3.568", "5.472", "2.832", "2.888", "2.336", "1.456", "0.288", "0.127", "0.657", "0.278", "1.225", "1.132", "24.983986", "25.185158", "26.05", "33.125", "30.875", "32.375", "31.875", "31.25", "40000", "-43.030043", "11.064009", "10", "1", "3/29/2022 11:47:34 AM", "P0033", "-1", "-1", "-1", "-1", "30 31 32 33", "1", "-1", "18.000000", "5.000000", "50.000000", "30.000000", "10.000000", "0.000000", "101", "0", "9", "REV-B_TETRA_RX-DVT-Quick_SN_P0033_032922-114225.csv"], ["25", "18.75", "3.000000", "5", "-73", "-1", "-1", "20.000000", "0.569196", "10.672434", "2", "0", "2", "2", "2", "2", "9.995", "10", "-41.791", "31.209", "9.965804", "-39.734641", "-57.177492", "17.442851", "9.965804", "12.613508", "18.311", "0.997", "0.996", "1.807", "3.316", "1.195", "4.992", "3.317", "2.498", "2.516", "3.568", "5.472", "2.824", "2.888", "2.336", "1.456", "0.284", "0.128", "0.686", "0.3", "1.227", "1.154", "24.982334", "25.244013", "27.1", "33.125", "31", "32.25", "32", "31.25", "20000", "-41.009443", "13.692614", "11", "1", "3/29/2022 11:47:48 AM", "P0033", "-1", "-1", "-1", "-1", "30 31 32 33", "1", "-1", "18.000000", "5.000000", "50.000000", "30.000000", "15.000000", "0.000000", "111", "1", "9", "REV-B_TETRA_RX-DVT-Quick_SN_P0033_032922-114225.csv"], ["25", "18.75", "3.000000", "5", "-73", "-1", "-1", "25.000000", "0.565884", "10.610327", "2", "0", "2", "2", "2", "2", "12.495", "10", "-34.544", "38.456", "9.965804", "-32.467577", "-56.90383", "24.436252", "9.965804", "5.64017", "18.311", "0.998", "0.994", "1.807", "3.316", "1.194", "4.99", "3.315", "2.498", "2.518", "3.568", "5.472", "2.832", "2.888", "2.336", "1.448", "0.29", "0.129", "0.668", "0.292", "1.226", "1.149", "24.981443", "25.186216", "27.1", "33.25", "31.125", "32.5", "32", "31.25", "25000", "-41.697643", "10.481807", "12", "1", "3/29/2022 11:47:58 AM", "P0033", "-1", "-1", "-1", "-1", "30 31 32 33", "1", "-1", "18.000000", "5.000000", "50.000000", "30.000000", "8.000000", "0.000000", "111", "1", "9", "REV-B_TETRA_RX-DVT-Quick_SN_P0033_032922-114225.csv"], ["25", "18.75", "3.000000", "5", "-73", "-1", "-1", "30.000000", "0.568936", "10.667548", "3", "0", "2", "2", "2", "2", "14.995", "10", "-36.579", "36.421", "9.965804", "-34.529812", "-59.478393", "24.948581", "9.965804", "5.100607", "18.32", "0.997", "0.996", "1.808", "3.318", "1.194", "4.99", "3.316", "2.497", "2.517", "3.568", "5.472", "2.824", "2.888", "2.336", "1.448", "0.288", "0.128", "0.689", "0.295", "1.226", "1.147", "24.978163", "25.18915", "28.15", "33", "31", "32.25", "32", "31.25", "30000", "-42.531268", "10.500729", "13", "1", "3/29/2022 11:48:09 AM", "P0033", "-1", "-1", "-1", "-1", "30 31 32 33", "1", "-1", "18.000000", "5.000000", "50.000000", "30.000000", "6.500000", "0.000000", "111", "1", "9", "REV-B_TETRA_RX-DVT-Quick_SN_P0033_032922-114225.csv"], ["25", "18.75", "3.000000", "5", "-73", "-1", "-1", "35.000000", "0.566788", "10.627281", "3", "0", "2", "2", "2", "2", "17.495", "10", "-43.405", "29.595", "9.965804", "-41.22646", "-63.599396", "22.372936", "9.965804", "7.805604", "18.32", "0.996", "0.995", "1.807", "3.315", "1.195", "4.993", "3.314", "2.497", "2.515", "3.568", "5.472", "2.824", "2.888", "2.336", "1.448", "0.284", "0.127", "0.684", "0.292", "1.226", "1.112", "24.98241", "25.189056", "28.15", "33.125", "31.125", "32.5", "32", "31.375", "35000", "-41.740204", "10.705545", "14", "1", "3/29/2022 11:48:19 AM", "P0033", "-1", "-1", "-1", "-1", "30 31 32 33", "1", "-1", "18.000000", "5.000000", "50.000000", "30.000000", "9.000000", "0.000000", "101", "0", "9", "REV-B_TETRA_RX-DVT-Quick_SN_P0033_032922-114225.csv"], ["25", "18.75", "3.000000", "5", "-73", "-1", "-1", "40.000000", "0.559835", "10.496908", "3", "0", "2", "2", "2", "2", "19.995", "10", "-45.892", "27.108", "9.965804", "-43.715005", "-66.201275", "22.486271", "9.965804", "7.690725", "18.329", "0.998", "0.995", "1.808", "3.315", "1.195", "4.99", "3.316", "2.499", "2.516", "3.568", "5.472", "2.832", "2.896", "2.336", "1.448", "0.282", "0.129", "0.657", "0.278", "1.226", "1.119", "25.036692", "25.130362", "27.1", "33", "31", "32.375", "32", "31.25", "40000", "-43.030043", "10.748362", "15", "1", "3/29/2022 11:48:30 AM", "P0033", "-1", "-1", "-1", "-1", "30 31 32 33", "1", "-1", "18.000000", "5.000000", "50.000000", "30.000000", "10.000000", "0.000000", "101", "0", "9", "REV-B_TETRA_RX-DVT-Quick_SN_P0033_032922-114225.csv"], ["25", "18.75", "4.000000", "5", "-73", "-1", "-1", "20.000000", "0.569984", "10.687207", "2", "0", "2", "2", "2", "2", "9.995", "10", "-40.021", "32.979", "9.965804", "-37.912785", "-56.529531", "18.616746", "9.965804", "11.491469", "18.293", "0.996", "0.996", "1.807", "3.316", "1.193", "4.992", "3.317", "2.496", "2.516", "3.568", "5.472", "2.824", "2.888", "2.336", "1.448", "0.289", "0.127", "0.686", "0.3", "1.226", "1.122", "25.093027", "25.250462", "27.1", "33.25", "31", "32.5", "32.25", "31.125", "20000", "-41.009443", "13.610743", "16", "1", "3/29/2022 11:48:44 AM", "P0033", "-1", "-1", "-1", "-1", "30 31 32 33", "1", "-1", "18.000000", "5.000000", "50.000000", "30.000000", "15.000000", "0.000000", "111", "1", "9", "REV-B_TETRA_RX-DVT-Quick_SN_P0033_032922-114225.csv"], ["25", "18.75", "4.000000", "5", "-73", "-1", "-1", "25.000000", "0.565701", "10.60689", "2", "0", "2", "2", "2", "2", "12.495", "10", "-33.558", "39.442", "9.965804", "-31.453021", "-56.199732", "24.746711", "9.965804", "5.358268", "18.32", "0.999", "0.996", "1.809", "3.316", "1.196", "4.99", "3.317", "2.497", "2.517", "3.568", "5.472", "2.832", "2.888", "2.336", "1.448", "0.282", "0.128", "0.669", "0.292", "1.226", "1.125", "25.034227", "25.191473", "27.1", "33.125", "31.125", "32.5", "32.125", "31.375", "25000", "-41.697643", "10.32326", "17", "1", "3/29/2022 11:48:54 AM", "P0033", "-1", "-1", "-1", "-1", "30 31 32 33", "1", "-1", "18.000000", "5.000000", "50.000000", "30.000000", "8.000000", "0.000000", "111", "1", "9", "REV-B_TETRA_RX-DVT-Quick_SN_P0033_032922-114225.csv"], ["25", "18.75", "4.000000", "5", "-73", "-1", "-1", "30.000000", "0.569667", "10.681251", "3", "0", "2", "2", "2", "2", "14.995", "10", "-36.871", "36.129", "9.965804", "-34.816471", "-59.611387", "24.794916", "9.965804", "5.259613", "18.311", "0.996", "0.995", "1.807", "3.315", "1.196", "4.99", "3.317", "2.496", "2.516", "3.568", "5.472", "2.824", "2.888", "2.336", "1.448", "0.29", "0.128", "0.688", "0.295", "1.226", "1.135", "25.033773", "25.189878", "28.15", "33.125", "31.125", "32.375", "32.125", "31.25", "30000", "-42.531268", "10.356341", "18", "1", "3/29/2022 11:49:04 AM", "P0033", "-1", "-1", "-1", "-1", "30 31 32 33", "1", "-1", "18.000000", "5.000000", "50.000000", "30.000000", "6.500000", "0.000000", "111", "1", "9", "REV-B_TETRA_RX-DVT-Quick_SN_P0033_032922-114225.csv"], ["25", "18.75", "4.000000", "5", "-73", "-1", "-1", "35.000000", "0.567024", "10.631707", "3", "0", "2", "2", "2", "2", "17.495", "10", "-42.439", "30.561", "9.965804", "-40.275433", "-63.414415", "23.138982", "9.965804", "7.024585", "18.311", "0.997", "0.994", "1.807", "3.314", "1.195", "4.99", "3.317", "2.496", "2.517", "3.568", "5.472", "2.832", "2.888", "2.336", "1.456", "0.288", "0.128", "0.683", "0.293", "1.225", "1.12", "25.08617", "25.183359", "27.1", "33.125", "31.125", "32.375", "32", "31.375", "35000", "-41.740204", "10.898454", "19", "1", "3/29/2022 11:49:15 AM", "P0033", "-1", "-1", "-1", "-1", "30 31 32 33", "1", "-1", "18.000000", "5.000000", "50.000000", "30.000000", "9.000000", "0.000000", "111", "1", "9", "REV-B_TETRA_RX-DVT-Quick_SN_P0033_032922-114225.csv"], ["25", "18.75", "4.000000", "5", "-73", "-1", "-1", "40.000000", "0.558596", "10.473666", "3", "0", "2", "2", "2", "2", "19.995", "10", "-45.617", "27.383", "9.965804", "-43.461601", "-65.824684", "22.363083", "9.965804", "7.792316", "18.329", "0.997", "0.996", "1.808", "3.315", "1.194", "4.992", "3.315", "2.498", "2.516", "3.568", "5.472", "2.832", "2.896", "2.336", "1.456", "0.288", "0.128", "0.657", "0.278", "1.225", "1.109", "25.031197", "25.187513", "27.1", "33.125", "31", "32.5", "32", "31.375", "40000", "-43.030043", "10.286318", "20", "1", "3/29/2022 11:49:26 AM", "P0033", "-1", "-1", "-1", "-1", "30 31 32 33", "1", "-1", "18.000000", "5.000000", "50.000000", "30.000000", "10.000000", "0.000000", "101", "0", "9", "REV-B_TETRA_RX-DVT-Quick_SN_P0033_032922-114225.csv"], ["25", "18.75", "5.000000", "5", "-73", "-1", "-1", "20.000000", "0.568759", "10.664233", "2", "0", "2", "2", "2", "2", "9.995", "10", "-40.401", "32.599", "9.965804", "-38.239629", "-56.65276", "18.413131", "9.965804", "11.74824", "18.311", "0.997", "0.995", "1.807", "3.315", "1.195", "4.992", "3.316", "2.498", "2.516", "3.568", "5.472", "2.824", "2.888", "2.336", "1.456", "0.288", "0.128", "0.686", "0.3", "1.225", "1.149", "24.959276", "25.241495", "27.1", "33", "31.125", "32.5", "32.125", "31.125", "20000", "-41.009443", "13.582175", "21", "1", "3/29/2022 11:49:39 AM", "P0033", "-1", "-1", "-1", "-1", "30 31 32 33", "1", "-1", "18.000000", "5.000000", "50.000000", "30.000000", "15.000000", "0.000000", "111", "1", "9", "REV-B_TETRA_RX-DVT-Quick_SN_P0033_032922-114225.csv"], ["25", "18.75", "5.000000", "5", "-73", "-1", "-1", "25.000000", "0.564387", "10.582251", "2", "0", "2", "2", "2", "2", "12.495", "10", "-34.486", "38.514", "9.965804", "-32.495831", "-56.909748", "24.413917", "9.965804", "5.576252", "18.32", "0.998", "0.994", "1.807", "3.316", "1.193", "4.992", "3.316", "2.498", "2.516", "3.568", "5.472", "2.832", "2.888", "2.336", "1.448", "0.282", "0.128", "0.669", "0.292", "1.225", "1.139", "25.023981", "25.185495", "27.1", "33.25", "31.125", "32.5", "32", "31.25", "25000", "-41.697643", "10.338612", "22", "1", "3/29/2022 11:49:50 AM", "P0033", "-1", "-1", "-1", "-1", "30 31 32 33", "1", "-1", "18.000000", "5.000000", "50.000000", "30.000000", "8.000000", "0.000000", "111", "1", "9", "REV-B_TETRA_RX-DVT-Quick_SN_P0033_032922-114225.csv"], ["25", "18.75", "5.000000", "5", "-73", "-1", "-1", "30.000000", "0.568503", "10.659439", "3", "0", "2", "2", "2", "2", "14.995", "10", "-36.257", "36.743", "9.965804", "-34.227624", "-59.03033", "24.802706", "9.965804", "5.22667", "18.311", "0.997", "0.995", "1.808", "3.316", "1.195", "4.99", "3.316", "2.497", "2.516", "3.568", "5.472", "2.824", "2.888", "2.336", "1.448", "0.282", "0.128", "0.689", "0.294", "1.226", "1.113", "25.015224", "25.179966", "28.15", "33.25", "31.25", "32.5", "32.125", "31.25", "30000", "-42.531268", "10.3116", "23", "1", "3/29/2022 11:50:00 AM", "P0033", "-1", "-1", "-1", "-1", "30 31 32 33", "1", "-1", "18.000000", "5.000000", "50.000000", "30.000000", "6.500000", "0.000000", "111", "1", "9", "REV-B_TETRA_RX-DVT-Quick_SN_P0033_032922-114225.csv"], ["25", "18.75", "5.000000", "5", "-73", "-1", "-1", "35.000000", "0.566003", "10.612558", "3", "0", "2", "2", "2", "2", "17.495", "10", "-42.197", "30.803", "9.965804", "-40.042527", "-62.132186", "22.089659", "9.965804", "8.064814", "18.311", "0.998", "0.996", "1.807", "3.315", "1.195", "4.992", "3.316", "2.496", "2.517", "3.568", "5.472", "2.824", "2.888", "2.336", "1.456", "0.288", "0.128", "0.684", "0.292", "1.226", "1.145", "25.013937", "25.181458", "28.15", "33.25", "31.25", "32.375", "32.125", "31.25", "35000", "-41.740204", "10.377699", "24", "1", "3/29/2022 11:50:10 AM", "P0033", "-1", "-1", "-1", "-1", "30 31 32 33", "1", "-1", "18.000000", "5.000000", "50.000000", "30.000000", "9.000000", "0.000000", "111", "1", "9", "REV-B_TETRA_RX-DVT-Quick_SN_P0033_032922-114225.csv"], ["25", "18.75", "5.000000", "5", "-73", "-1", "-1", "40.000000", "0.558588", "10.473525", "3", "0", "2", "2", "2", "2", "19.995", "10", "-45.624", "27.376", "9.965804", "-43.466521", "-65.070224", "21.603703", "9.965804", "8.553776", "18.311", "0.996", "0.994", "1.807", "3.315", "1.194", "4.989", "3.315", "2.498", "2.518", "3.568", "5.472", "2.832", "2.888", "2.336", "1.456", "0.282", "0.128", "0.657", "0.278", "1.225", "1.135", "25.010406", "25.240318", "26.05", "33.25", "31", "32.5", "32.125", "31.375", "40000", "-43.030043", "10.290322", "25", "1", "3/29/2022 11:50:21 AM", "P0033", "-1", "-1", "-1", "-1", "30 31 32 33", "1", "-1", "18.000000", "5.000000", "50.000000", "30.000000", "10.000000", "0.000000", "101", "0", "9", "REV-B_TETRA_RX-DVT-Quick_SN_P0033_032922-114225.csv"], ["25", "18.75", "6.000000", "5", "-73", "-1", "-1", "20.000000", "0.567979", "10.649612", "2", "0", "2", "2", "2", "2", "9.995", "10", "-39.876", "33.124", "9.965804", "-37.689382", "-56.766567", "19.077185", "9.965804", "11.109433", "18.32", "0.996", "0.996", "1.808", "3.317", "1.196", "4.99", "3.314", "2.496", "2.517", "3.568", "5.472", "2.824", "2.888", "2.336", "1.456", "0.284", "0.128", "0.685", "0.3", "1.225", "1.136", "25.006052", "25.180799", "28.15", "33.125", "31.125", "32.5", "32.25", "31.375", "20000", "-41.009443", "13.656313", "26", "1", "3/29/2022 11:50:34 AM", "P0033", "-1", "-1", "-1", "-1", "30 31 32 33", "1", "-1", "18.000000", "5.000000", "50.000000", "30.000000", "15.000000", "0.000000", "111", "1", "9", "REV-B_TETRA_RX-DVT-Quick_SN_P0033_032922-114225.csv"], ["25", "18.75", "6.000000", "5", "-73", "-1", "-1", "25.000000", "0.56491", "10.592068", "2", "0", "2", "2", "2", "2", "12.495", "10", "-34.01", "38.99", "9.965804", "-31.871954", "-55.985571", "24.113616", "9.965804", "6.024429", "18.329", "0.996", "0.994", "1.807", "3.315", "1.193", "4.993", "3.317", "2.496", "2.516", "3.568", "5.472", "2.832", "2.888", "2.336", "1.448", "0.284", "0.128", "0.668", "0.292", "1.225", "1.113", "25.014597", "25.185217", "27.1", "33.375", "31.25", "32.5", "32.125", "31.375", "25000", "-41.697643", "10.37923", "27", "1", "3/29/2022 11:50:45 AM", "P0033", "-1", "-1", "-1", "-1", "30 31 32 33", "1", "-1", "18.000000", "5.000000", "50.000000", "30.000000", "8.000000", "0.000000", "111", "1", "9", "REV-B_TETRA_RX-DVT-Quick_SN_P0033_032922-114225.csv"], ["25", "18.75", "6.000000", "5", "-73", "-1", "-1", "30.000000", "0.567354", "10.637895", "3", "0", "2", "2", "2", "2", "14.995", "10", "-37.283", "35.717", "9.965804", "-35.186326", "-60.015322", "24.828996", "9.965804", "5.267678", "18.32", "0.996", "0.996", "1.808", "3.315", "1.195", "4.992", "3.317", "2.498", "2.517", "3.568", "5.472", "2.824", "2.888", "2.336", "1.448", "0.29", "0.129", "0.688", "0.295", "1.226", "1.106", "25.006163", "25.179977", "28.15", "33.25", "31", "32.5", "32.25", "31.25", "30000", "-42.531268", "10.365277", "28", "1", "3/29/2022 11:50:55 AM", "P0033", "-1", "-1", "-1", "-1", "30 31 32 33", "1", "-1", "18.000000", "5.000000", "50.000000", "30.000000", "6.500000", "0.000000", "111", "1", "9", "REV-B_TETRA_RX-DVT-Quick_SN_P0033_032922-114225.csv"], ["25", "18.75", "6.000000", "5", "-73", "-1", "-1", "35.000000", "0.565674", "10.60638", "3", "0", "2", "2", "2", "2", "17.495", "10", "-41.248", "31.752", "9.965804", "-38.992964", "-62.000115", "23.007151", "9.965804", "7.247885", "18.311", "0.997", "0.994", "1.807", "3.315", "1.194", "4.99", "3.317", "2.497", "2.518", "3.568", "5.472", "2.832", "2.888", "2.336", "1.456", "0.284", "0.129", "0.683", "0.292", "1.224", "1.115", "24.951511", "25.182125", "28.15", "33.25", "31.125", "32.625", "32", "31.375", "35000", "-41.740204", "10.28063", "29", "1", "3/29/2022 11:51:05 AM", "P0033", "-1", "-1", "-1", "-1", "30 31 32 33", "1", "-1", "18.000000", "5.000000", "50.000000", "30.000000", "9.000000", "0.000000", "111", "1", "9", "REV-B_TETRA_RX-DVT-Quick_SN_P0033_032922-114225.csv"], ["25", "18.75", "6.000000", "5", "-73", "-1", "-1", "40.000000", "0.559541", "10.491401", "3", "0", "2", "2", "2", "2", "19.995", "10", "-45.525", "27.475", "9.965804", "-43.40969", "-64.476696", "21.067006", "9.965804", "9.048304", "18.329", "0.996", "0.996", "1.807", "3.316", "1.195", "4.992", "3.317", "2.498", "2.515", "3.568", "5.472", "2.832", "2.896", "2.336", "1.456", "0.288", "0.128", "0.657", "0.279", "1.225", "1.117", "24.952892", "25.180176", "26.05", "33.25", "31", "32.5", "32.125", "31.25", "40000", "-43.030043", "10.361334", "30", "1", "3/29/2022 11:51:16 AM", "P0033", "-1", "-1", "-1", "-1", "30 31 32 33", "1", "-1", "18.000000", "5.000000", "50.000000", "30.000000", "10.000000", "0.000000", "101", "0", "9", "REV-B_TETRA_RX-DVT-Quick_SN_P0033_032922-114225.csv"], ["25", "18.75", "7.000000", "5", "-73", "-1", "-1", "20.000000", "0.569671", "10.681324", "2", "0", "2", "2", "2", "2", "9.995", "10", "-40.815", "32.185", "9.965804", "-38.665384", "-56.780314", "18.11493", "9.965804", "12.034686", "18.311", "0.996", "0.996", "1.807", "3.316", "1.195", "4.995", "3.314", "2.496", "2.518", "3.568", "5.472", "2.824", "2.888", "2.336", "1.448", "0.282", "0.127", "0.686", "0.3", "1.226", "1.127", "24.953074", "25.179266", "27.1", "33.375", "31.25", "32.375", "32.25", "31.25", "20000", "-41.009443", "13.584268", "31", "1", "3/29/2022 11:51:29 AM", "P0033", "-1", "-1", "-1", "-1", "30 31 32 33", "1", "-1", "18.000000", "5.000000", "50.000000", "30.000000", "15.000000", "0.000000", "111", "1", "9", "REV-B_TETRA_RX-DVT-Quick_SN_P0033_032922-114225.csv"], ["25", "18.75", "7.000000", "5", "-73", "-1", "-1", "25.000000", "0.565739", "10.607599", "2", "0", "2", "2", "2", "2", "12.495", "10", "-35.054", "37.946", "9.965804", "-33.063722", "-57.302932", "24.23921", "9.965804", "5.751068", "18.32", "0.996", "0.996", "1.807", "3.316", "1.195", "4.992", "3.316", "2.498", "2.516", "3.568", "5.472", "2.832", "2.888", "2.336", "1.456", "0.288", "0.128", "0.669", "0.292", "1.228", "1.159", "24.952223", "25.229593", "27.1", "33.25", "31.25", "32.625", "32.125", "31.375", "25000", "-41.697643", "10.307795", "32", "1", "3/29/2022 11:51:40 AM", "P0033", "-1", "-1", "-1", "-1", "30 31 32 33", "1", "-1", "18.000000", "5.000000", "50.000000", "30.000000", "8.000000", "0.000000", "111", "1", "9", "REV-B_TETRA_RX-DVT-Quick_SN_P0033_032922-114225.csv"], ["25", "18.75", "7.000000", "5", "-73", "-1", "-1", "30.000000", "0.568261", "10.654898", "3", "0", "2", "2", "2", "2", "14.995", "10", "-36.264", "36.736", "9.965804", "-34.133015", "-59.415787", "25.282772", "9.965804", "4.848213", "18.329", "0.997", "0.996", "1.807", "3.314", "1.194", "4.99", "3.317", "2.496", "2.516", "3.568", "5.472", "2.824", "2.888", "2.336", "1.448", "0.283", "0.128", "0.689", "0.295", "1.225", "1.117", "24.950842", "25.228264", "28.15", "33.25", "31.125", "32.625", "32.125", "31.375", "30000", "-42.531268", "10.490804", "33", "1", "3/29/2022 11:51:50 AM", "P0033", "-1", "-1", "-1", "-1", "30 31 32 33", "1", "-1", "18.000000", "5.000000", "50.000000", "30.000000", "6.500000", "0.000000", "111", "1", "9", "REV-B_TETRA_RX-DVT-Quick_SN_P0033_032922-114225.csv"], ["25", "18.75", "7.000000", "5", "-73", "-1", "-1", "35.000000", "0.567675", "10.643908", "3", "0", "2", "2", "2", "2", "17.495", "10", "-42.534", "30.466", "9.965804", "-40.439073", "-63.069629", "22.630556", "9.965804", "7.464371", "18.311", "0.996", "0.995", "1.807", "3.315", "1.195", "4.99", "3.315", "2.496", "2.516", "3.568", "5.472", "2.824", "2.888", "2.336", "1.448", "0.288", "0.128", "0.684", "0.292", "1.226", "1.114", "24.896477", "25.16938", "27.1", "33.25", "31.25", "32.625", "32.125", "31.375", "35000", "-41.740204", "10.569302", "34", "1", "3/29/2022 11:52:01 AM", "P0033", "-1", "-1", "-1", "-1", "30 31 32 33", "1", "-1", "18.000000", "5.000000", "50.000000", "30.000000", "9.000000", "0.000000", "111", "1", "9", "REV-B_TETRA_RX-DVT-Quick_SN_P0033_032922-114225.csv"], ["25", "18.75", "7.000000", "5", "-73", "-1", "-1", "40.000000", "0.559448", "10.489652", "3", "0", "2", "2", "2", "2", "19.995", "10", "-46.551", "26.449", "9.965804", "-44.613001", "-66.004291", "21.39129", "9.965804", "8.546709", "18.329", "0.997", "0.996", "1.807", "3.316", "1.194", "4.993", "3.315", "2.497", "2.516", "3.568", "5.472", "2.832", "2.888", "2.336", "1.456", "0.282", "0.127", "0.657", "0.278", "1.225", "1.136", "24.957314", "25.16938", "27.1", "33.125", "31.125", "32.625", "31.875", "31.375", "40000", "-43.030043", "10.409809", "35", "1", "3/29/2022 11:52:11 AM", "P0033", "-1", "-1", "-1", "-1", "30 31 32 33", "1", "-1", "18.000000", "5.000000", "50.000000", "30.000000", "10.000000", "0.000000", "101", "0", "9", "REV-B_TETRA_RX-DVT-Quick_SN_P0033_032922-114225.csv"], ["25", "18.75", "8.000000", "5", "-73", "-1", "-1", "20.000000", "0.568566", "10.660607", "2", "0", "2", "2", "2", "2", "9.995", "10", "-40.849", "32.151", "9.965804", "-38.818566", "-56.347075", "17.528509", "9.965804", "12.501925", "18.311", "0.998", "0.995", "1.807", "3.315", "1.195", "4.992", "3.315", "2.496", "2.516", "3.568", "5.472", "2.824", "2.888", "2.336", "1.448", "0.284", "0.128", "0.686", "0.3", "1.226", "1.117", "25.019802", "25.228247", "27.1", "33.25", "31.125", "32.625", "32.125", "31.375", "20000", "-41.009443", "13.716725", "36", "1", "3/29/2022 11:52:25 AM", "P0033", "-1", "-1", "-1", "-1", "30 31 32 33", "1", "-1", "18.000000", "5.000000", "50.000000", "30.000000", "15.000000", "0.000000", "111", "1", "9", "REV-B_TETRA_RX-DVT-Quick_SN_P0033_032922-114225.csv"], ["25", "18.75", "8.000000", "5", "-73", "-1", "-1", "25.000000", "0.565711", "10.607083", "2", "0", "2", "2", "2", "2", "12.495", "10", "-34.8", "38.2", "9.965804", "-32.769672", "-57.008907", "24.239235", "9.965804", "5.791093", "18.329", "0.997", "0.995", "1.807", "3.314", "1.194", "4.993", "3.317", "2.496", "2.516", "3.568", "5.472", "2.832", "2.888", "2.336", "1.448", "0.282", "0.128", "0.669", "0.292", "1.228", "1.128", "25.022074", "25.22739", "27.1", "33.25", "31.25", "32.625", "32", "31.25", "25000", "-41.697643", "10.948414", "37", "1", "3/29/2022 11:52:36 AM", "P0033", "-1", "-1", "-1", "-1", "30 31 32 33", "1", "-1", "18.000000", "5.000000", "50.000000", "30.000000", "8.000000", "0.000000", "111", "1", "9", "REV-B_TETRA_RX-DVT-Quick_SN_P0033_032922-114225.csv"], ["25", "18.75", "8.000000", "5", "-73", "-1", "-1", "30.000000", "0.569299", "10.674366", "3", "0", "2", "2", "2", "2", "14.995", "10", "-36.661", "36.339", "9.965804", "-34.535792", "-59.050958", "24.515167", "9.965804", "5.610042", "18.302", "0.998", "0.995", "1.807", "3.316", "1.195", "4.989", "3.314", "2.498", "2.515", "3.568", "5.472", "2.824", "2.888", "2.336", "1.456", "0.29", "0.128", "0.688", "0.295", "1.226", "1.114", "25.021591", "25.230801", "28.15", "33.375", "31.25", "32.5", "32.25", "31.5", "30000", "-42.531268", "10.472914", "38", "1", "3/29/2022 11:52:46 AM", "P0033", "-1", "-1", "-1", "-1", "30 31 32 33", "1", "-1", "18.000000", "5.000000", "50.000000", "30.000000", "6.500000", "0.000000", "111", "1", "9", "REV-B_TETRA_RX-DVT-Quick_SN_P0033_032922-114225.csv"], ["25", "18.75", "8.000000", "5", "-73", "-1", "-1", "35.000000", "0.566667", "10.625016", "3", "0", "2", "2", "2", "2", "17.495", "10", "-43.481", "29.519", "9.965804", "-41.42763", "-63.649674", "22.222044", "9.965804", "7.831326", "18.32", "0.996", "0.996", "1.806", "3.314", "1.195", "4.993", "3.315", "2.497", "2.516", "3.568", "5.472", "2.824", "2.888", "2.336", "1.448", "0.284", "0.128", "0.684", "0.292", "1.225", "1.108", "25.019392", "25.230145", "28.15", "33.125", "31.25", "32.625", "32.25", "31.375", "35000", "-41.740204", "10.598635", "39", "1", "3/29/2022 11:52:57 AM", "P0033", "-1", "-1", "-1", "-1", "30 31 32 33", "1", "-1", "18.000000", "5.000000", "50.000000", "30.000000", "9.000000", "0.000000", "101", "0", "9", "REV-B_TETRA_RX-DVT-Quick_SN_P0033_032922-114225.csv"], ["25", "18.75", "8.000000", "5", "-73", "-1", "-1", "40.000000", "0.558543", "10.472679", "3", "0", "2", "2", "2", "2", "19.995", "10", "-46.351", "26.649", "9.965804", "-44.220796", "-65.350936", "21.13014", "9.965804", "9.000064", "18.32", "0.996", "0.995", "1.807", "3.315", "1.195", "4.99", "3.317", "2.497", "2.517", "3.568", "5.472", "2.832", "2.896", "2.336", "1.456", "0.284", "0.128", "0.657", "0.278", "1.224", "1.101", "25.08005", "25.225355", "27.1", "33.375", "31", "32.5", "32.125", "31.375", "40000", "-43.030043", "10.739114", "40", "1", "3/29/2022 11:53:08 AM", "P0033", "-1", "-1", "-1", "-1", "30 31 32 33", "1", "-1", "18.000000", "5.000000", "50.000000", "30.000000", "10.000000", "0.000000", "101", "0", "9", "REV-B_TETRA_RX-DVT-Quick_SN_P0033_032922-114225.csv"]]
  out "Header":string[][](array[string])
  in  "Header Row":i32=81
  in  "Header Column":i32=78
  out "all rows":string[][](array[string])
  out "error out":errorcluster
  in  "error in":errorcluster
  out "FirstFile":path=path "C:/RageATE Results/Files to Process/REV-B_TETRA_RX-DVT-Quick_SN_0033_032922-100611.csv"
  out "Output Path":path=path "C:/RageATE Results/Files to Process/REV-B_TETRA_RX-DVT-Quick_SN_0033_032922-100611_Concat.csv"
  out "path out":path=path "C:/RageATE Results/Files to Process"
  out "filenames":string[](array[string])=["REV-B_TETRA_RX-DVT-Quick_SN_0033_032922-100611.csv", "REV-B_TETRA_RX-DVT-Quick_SN_P0033_032922-101720.csv", "REV-B_TETRA_RX-DVT-Quick_SN_P0033_032922-102756.csv", "REV-B_TETRA_RX-DVT-Quick_SN_P0033_032922-103832.csv", "REV-B_TETRA_RX-DVT-Quick_SN_P0033_032922-104907.csv", "REV-B_TETRA_RX-DVT-Quick_SN_P0033_032922-105945.csv", "REV-B_TETRA_RX-DVT-Quick_SN_P0033_032922-111019.csv", "REV-B_TETRA_RX-DVT-Quick_SN_P0033_032922-112059.csv", "REV-B_TETRA_RX-DVT-Quick_SN_P0033_032922-113139.csv", "REV-B_TETRA_RX-DVT-Quick_SN_P0033_032922-114225.csv"]
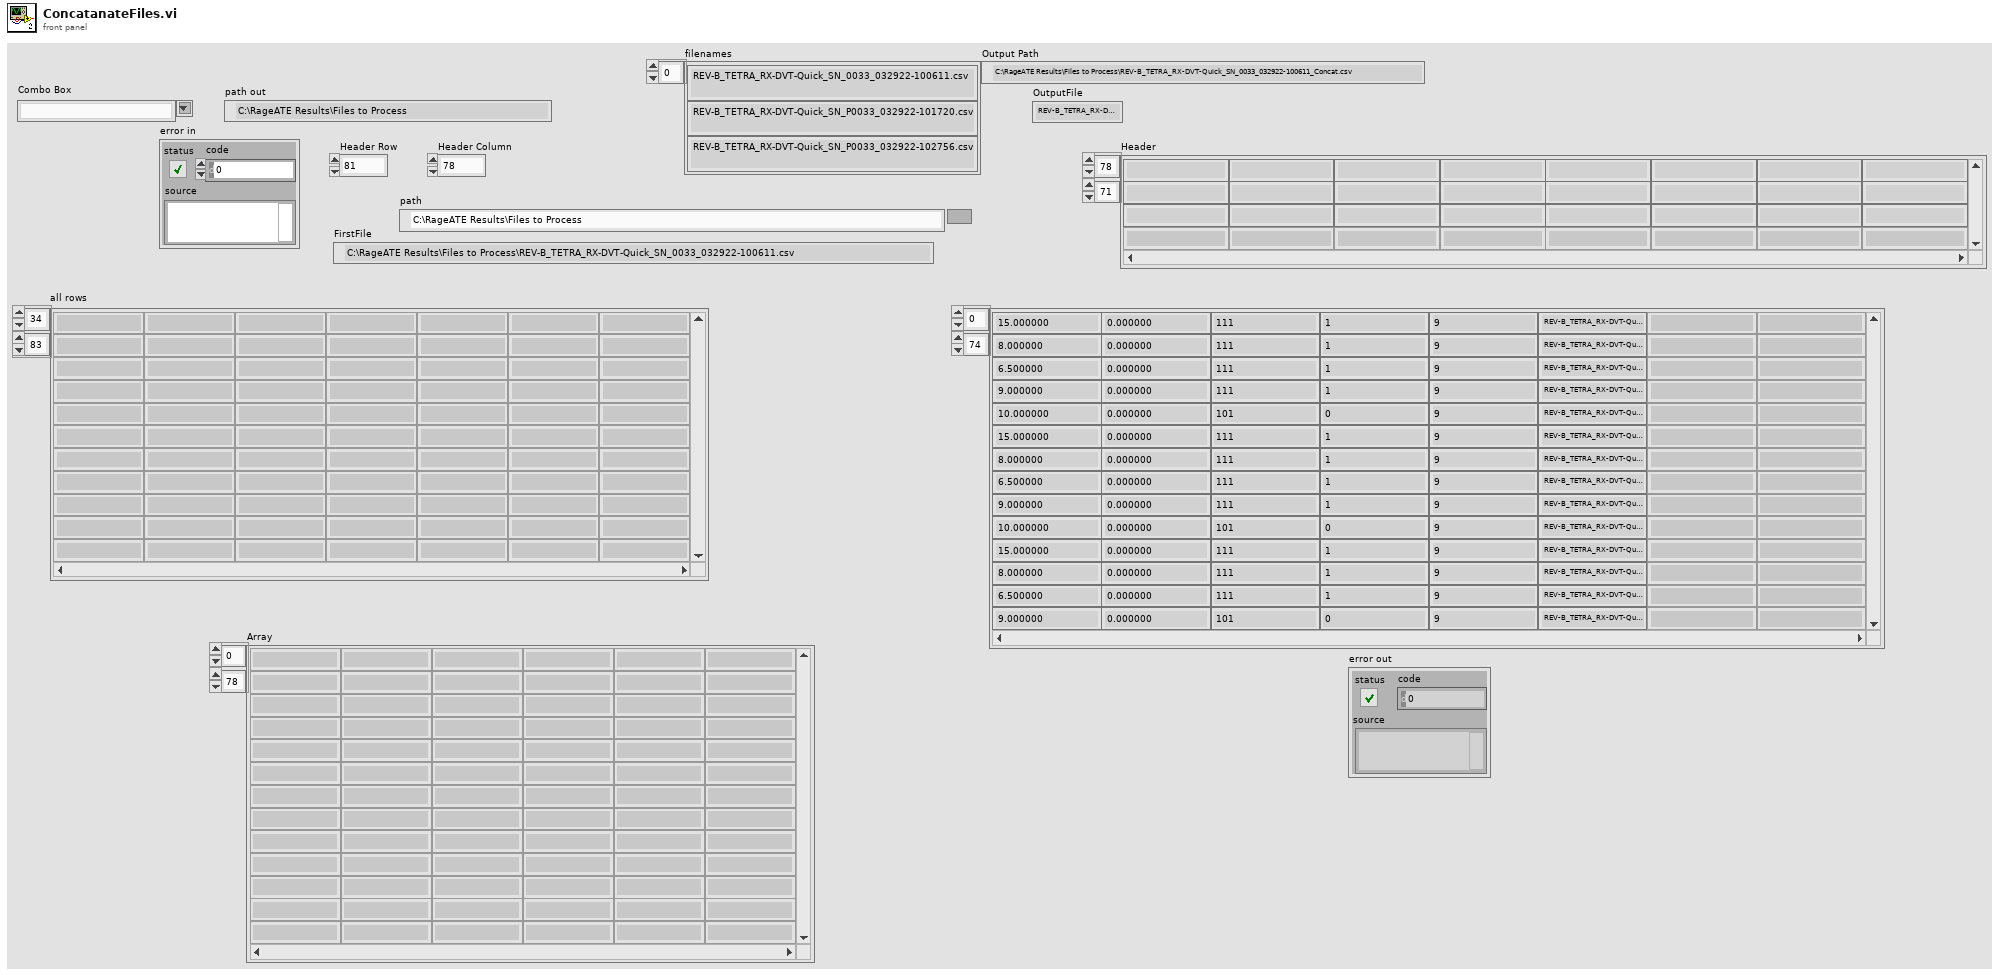
[diagram p1: front panel]
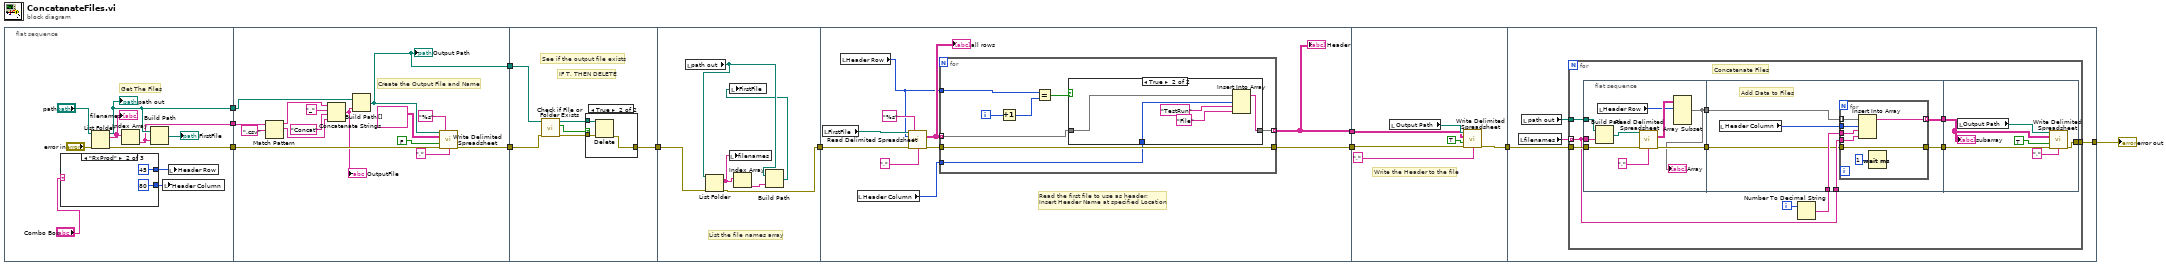
[diagram p0: block diagram]
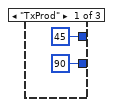
[diagram p2: hidden frame]
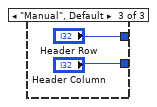
[diagram p3: hidden frame]
diagram:
  n1 = flat-sequence {
    tunnel: [w19] -> w11
    tunnel: [w18] -> w10
    tunnel: [w15] -> w9
    tunnel: [w37] -> w5
    tunnel: w9 -> [w42]
    tunnel: w10 -> [w35]
    tunnel: w11 -> [w36]
    tunnel: [w28] -> w4
    tunnel: w5 -> [w47]
    tunnel: [w45] -> w3
    tunnel: w4 -> [w48]
    tunnel: w3 -> [w57]
    tunnel: [w53] -> w2
    tunnel: w2 -> [w66]
    tunnel: [w62] -> w8
    tunnel: [w61] -> w7
    tunnel: w8 -> [w85]
    tunnel: w7 -> [w84]
    tunnel: [w83] -> w6
    tunnel: w6 -> [w92]
    tunnel: [w89] -> w1
    frame #0 {
      # "Get The Files"
      n2 = case shown="\"RxProd\"" "Combo Box" {
        tunnel: [45 ("Header Row") 45 ("Header Row") "Header Row"] -> w14
        tunnel: [90 ("Header Column") 80 ("Header Column") "Header Column"] -> w13
        frame "TxProd" {
        }
        frame "RxProd" {
        }
        frame "Manual", Default {
        }
      }
      n3 = List Folder(path="path", error in="error in") -> (path out=w19:path, filenames=w20:string[], error out=w15:errorcluster)  [unwired: 2 in, 1 out]
      "filenames" <- w20
      "path out" <- w19
      n4 = Index Array(array=w20) -> (element=w18:string)  [unwired: 1 in]
      n5 = Build Path(base path=w19, name or relative path=w18) -> (appended path=→"FirstFile":path)
      n6 = local write "Header Column"(w13) -> ()
      n7 = local write "Header Row"(w14) -> ()
    }
    frame #1 {
      # "Create the Output File and Name"
      n8 = Match Pattern(string=w35, regular expression=".csv") -> (before substring=w32:string, match substring=w29:string)  [unwired: 1 in, 2 out]
      n9 = Concatenate Strings(w32, "_" ("string"), "Concat" ("string"), w29) -> (w33:string)
      "OutputFile" <- w33
      n10 = Build Path(base path=w36, name or relative path=w33) -> (appended path=w28:path)
      "Output Path" <- w28
      n11 = call-poly <vilib>:"Write Delimited Spreadsheet.vi"("file path (dialog if empty)"=w28, "format (%s)"="%s" ("format (%.3f)"), "2D data"=string[][] [], "append to file? (new file:F)"=FALSE, "error in (no error)"=w42, "delimiter (\\t)"="," ("delimiter (\\t)")) -> ("error out"=w37:errorcluster)  [unwired: 8 in, 1 out]
    }
    frame #2 {
      # "IF T, THEN DELETE"
      # "See if the output file exists"
      n12 = call <vilib>:"Check if File or Folder Exists.vi"("error in (no error)"=w47, "path"=w48) -> ("error out"=w46:errorcluster, "file or folder exists?"=w43:bool, "dup path"=w44:path)  [unwired: 7 in]
      n13 = case shown="True" w43 {
        tunnel: w46 -> [w49 w52]
        tunnel: [w49 w51] -> w45
        tunnel: w44 -> [_ w50]
        frame False {
        }
        frame True {
          n14 = Delete(path (use dialog)=w50, error in=w52) -> (error out=w51:errorcluster)  [unwired: 3 in, 2 out]
        }
      }
    }
    frame #3 {
      # "List the file names array"
      n15 = local read "path out"() -> (w55:path)
      n16 = List Folder(path=w55, error in=w57) -> (filenames=w56:string[], error out=w53:errorcluster)  [unwired: 2 in, 2 out]
      n17 = local write "filenames"(w56) -> ()
      n18 = Index Array(array=w56) -> (element=w58:string)  [unwired: 1 in]
      n19 = Build Path(base path=w55, name or relative path=w58) -> (appended path=w54:path)
      n20 = local write "FirstFile"(w54) -> ()
    }
    frame #4 {
      # "Read the first file to use as header;\nInsert Header Name at specified Location"
      n21 = local read "FirstFile"() -> (w68:path)
      n22 = local read "Header Row"() -> (w60:i32)
      n23 = local read "Header Column"() -> (w59:i32)
      n24 = call-poly <vilib>:"Read Delimited Spreadsheet.vi"("file path (dialog if empty)"=w68, "format (%s)"="%s" ("format (%.3f)"), "number of rows (all:-1)"=w60, "error in (no error)"=w66, "delimiter (\\t)"="," ("delimiter (\\t)")) -> ("all rows"=w64:string[][], "error out"=w63:errorcluster)  [unwired: 5 in, 4 out]
      "all rows" <- w64
      n25 = for {
        tunnel: w64 -> [w76] mode=indexing
        tunnel: [w75] -> w61 mode=indexing
        tunnel: [w72] -> w62
        tunnel: w63 -> [w72]
        tunnel: w60 -> [w71]
        tunnel: w59 -> [w69]
        i -> [w74]
        n26 = Increment(x=w74) -> (x+1=w70:i32)
        n27 = Equal?(x=w71, y=w70) -> (x = y?=w73:bool)
        n28 = case shown="True" w73 {
          tunnel: w76 -> [w77 w82]
          tunnel: [w77 w81] -> w75
          tunnel: w69 -> [_ w78]
          frame False {
          }
          frame True {
            n29 = Insert Into Array(array=w82, index=w78, new element #1="TestRun" ("Insert Header"), new element #2="File" ("Insert Header")) -> (w81:string[])
          }
        }
      }
      "Header" <- w61
    }
    frame #5 {
      # "Write the Header to the file"
      n30 = local read "Output Path"() -> (w88:path)
      n31 = call-poly <vilib>:"Write Delimited Spreadsheet.vi"("file path (dialog if empty)"=w88, "2D data"=w84, "append to file? (new file:F)"=TRUE, "error in (no error)"=w85, "delimiter (\\t)"="," ("delimiter (\\t)")) -> ("error out"=w83:errorcluster)  [unwired: 9 in, 1 out]
    }
    frame #6 {
      n32 = local read "filenames"() -> (w91:string[])
      n33 = local read "path out"() -> (w90:path)
      n34 = for {
        tunnel: w92 -> [w102]
        tunnel: w91 -> [w96] mode=indexing
        tunnel: w90 -> [w101]
        tunnel: [w93] -> w89
        i -> [w100]
        # "Concatenate Files"
        n35 = flat-sequence {
          tunnel: w102 -> [w111]
          tunnel: w101 -> [w110]
          tunnel: w96 -> [w109]
          tunnel: [w104] -> w99
          tunnel: [w108] -> w98
          tunnel: w99 -> [w118]
          tunnel: w98 -> [w114]
          tunnel: w97 -> [w116]
          tunnel: w96 -> [w115]
          tunnel: [w113] -> w95
          tunnel: [w112] -> w94
          tunnel: w95 -> [w130]
          tunnel: w94 -> [w128]
          tunnel: [w126] -> w93
          frame #0 {
            n36 = Build Path(base path=w110, name or relative path=w109) -> (appended path=w105:path)
            n37 = local read "Header Row"() -> (w103:i32)
            n38 = call-poly <vilib>:"Read Delimited Spreadsheet.vi"("file path (dialog if empty)"=w105, "error in (no error)"=w111, "delimiter (\\t)"="," ("delimiter (\\t)")) -> ("all rows"=w106:string[][], "error out"=w108:errorcluster)  [unwired: 7 in, 4 out]
            n39 = Array Subset(array=w106, index (row)=w103) -> (w104:string[][])  [unwired: 3 in]
            "Array" <- w104
          }
          frame #1 {
            # "Add Data to Files"
            n40 = local read "Header Column"() -> (w117:i32)
            n41 = for {
              tunnel: w118 -> [w125] mode=indexing
              tunnel: w117 -> [w124]
              tunnel: [w123] -> w113 mode=indexing
              tunnel: w116 -> [w122]
              tunnel: w115 -> [w121]
              tunnel: w114 -> [w120]
              tunnel: [w120] -> w112
              n42 = Insert Into Array(array=w125, index=w124, new element #1=w122, new element #2=w121) -> (w123:string[])
              n43 = Wait (ms)(milliseconds to wait=u32 1) -> ()  [unwired: 1 out]
            }
          }
          frame #2 {
            n44 = local read "Output Path"() -> (w131:path)
            n45 = call-poly <vilib>:"Write Delimited Spreadsheet.vi"("file path (dialog if empty)"=w131, "2D data"=w130, "append to file? (new file:F)"=TRUE, "error in (no error)"=w128, "delimiter (\\t)"="," ("delimiter (\\t)")) -> ("error out"=w126:errorcluster)  [unwired: 9 in, 1 out]
            "subarray" <- w130
          }
        }
        n46 = Number To Decimal String(number=w100) -> (decimal integer string=w97:string)  [unwired: 1 in]
      }
    }
  }
  "error out" <- w1
